vi "Set Call Status.vi"(8 "error in":errorcluster, 9 "Details":string, 10 "Status Code":T2=enum."INTERNAL", 11 "gRPCid in":T1) -> (0 "error out":errorcluster, 3 "gRPCid out":T1)   [LabVIEW 2019, in "grpc-lvsupport.lvlib"]
uses:
  grpc-lvsupport.lvlib
  typeDefs/gRPC Status Code.ctl
  Shared/grpcId.ctl
  <vilib>/Utility/error.llb/Error Cluster From Error Code.vi
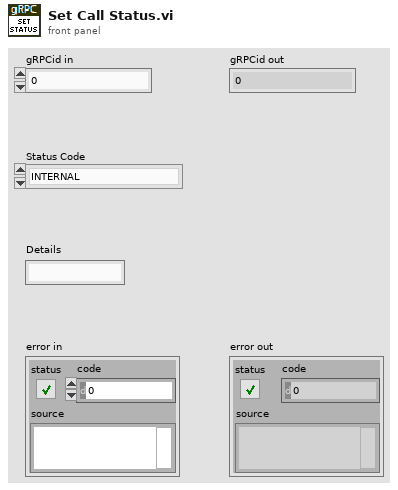
[diagram p1: front panel]
types:
  T1 = typedef "grpc-lvsupport.lvlib/grpcId.ctl" = u64
  T2 = typedef "grpc-lvsupport.lvlib/gRPC Status Code.ctl" = enum16{"OK", "CANCELLED", "UNKNOWN", "INVALID_ARGUMENT", "DEADLINE_EXCEEDED", "NOT_FOUND", "ALREADY_EXISTS", "PERMISSION_DENIED", "RESOURCE_EXHAUSTED", "FAILED_PRECONDITION", "ABORTED", "OUT_OF_RANGE", "UNIMPLEMENTED", "INTERNAL", "UNAVAILABLE", "DATA_LOSS", "UNAUTHENTICATED"}
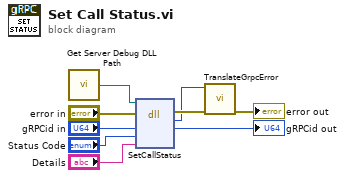
[diagram p0: block diagram]
diagram:
  n1 = call "Get Server Debug DLL Path.vi"() -> ("Server dll path"=w6:path)
  n2 = dll-call lib="?" fn="SetCallStatus"(path in=w6, error in="error in", "grpcId"="gRPCid in", "errorCode"="Status Code", "errorMessage"="Details") -> (error out=w8:errorcluster, "return type"=w5:i32, "grpcId"=→"gRPCid out":T1)  [unwired: 3 in, 1 out]
  n3 = call "TranslateGrpcError.vi"("error in"=w8, "Error Code"=w5) -> ("error out"=→"error out":errorcluster)  [unwired: 9 in]
